vi "测试1005.vi"() -> ()   [LabVIEW 2016]
uses:
  <vilib>/Instr/_visa.llb/VISA Configure Serial Port (Instr).vi
panel:
  out "发送命令 2":string
  in  "暂停 2":bool
  in  "故障腿 2":string(combo)
  in  "控制方法 2":string(combo)
  in  "退化故障 2":string(combo)
  in  "卡滞角度 2":string
  in  "角度（小数） 2":string
  in  "卡滞发生时间 2":string
  in  "小数 2":string
  in  "控制程序启动 2":bool
  in  "复位 2":bool
  out "接受字符串":string
  in  "波特率":dbl
  in  "data bits (8)":u16=8 caption="数据比特(8)" min=5 max=8 step=1
  in  "arduino端口":refnum<visa-resource-name>
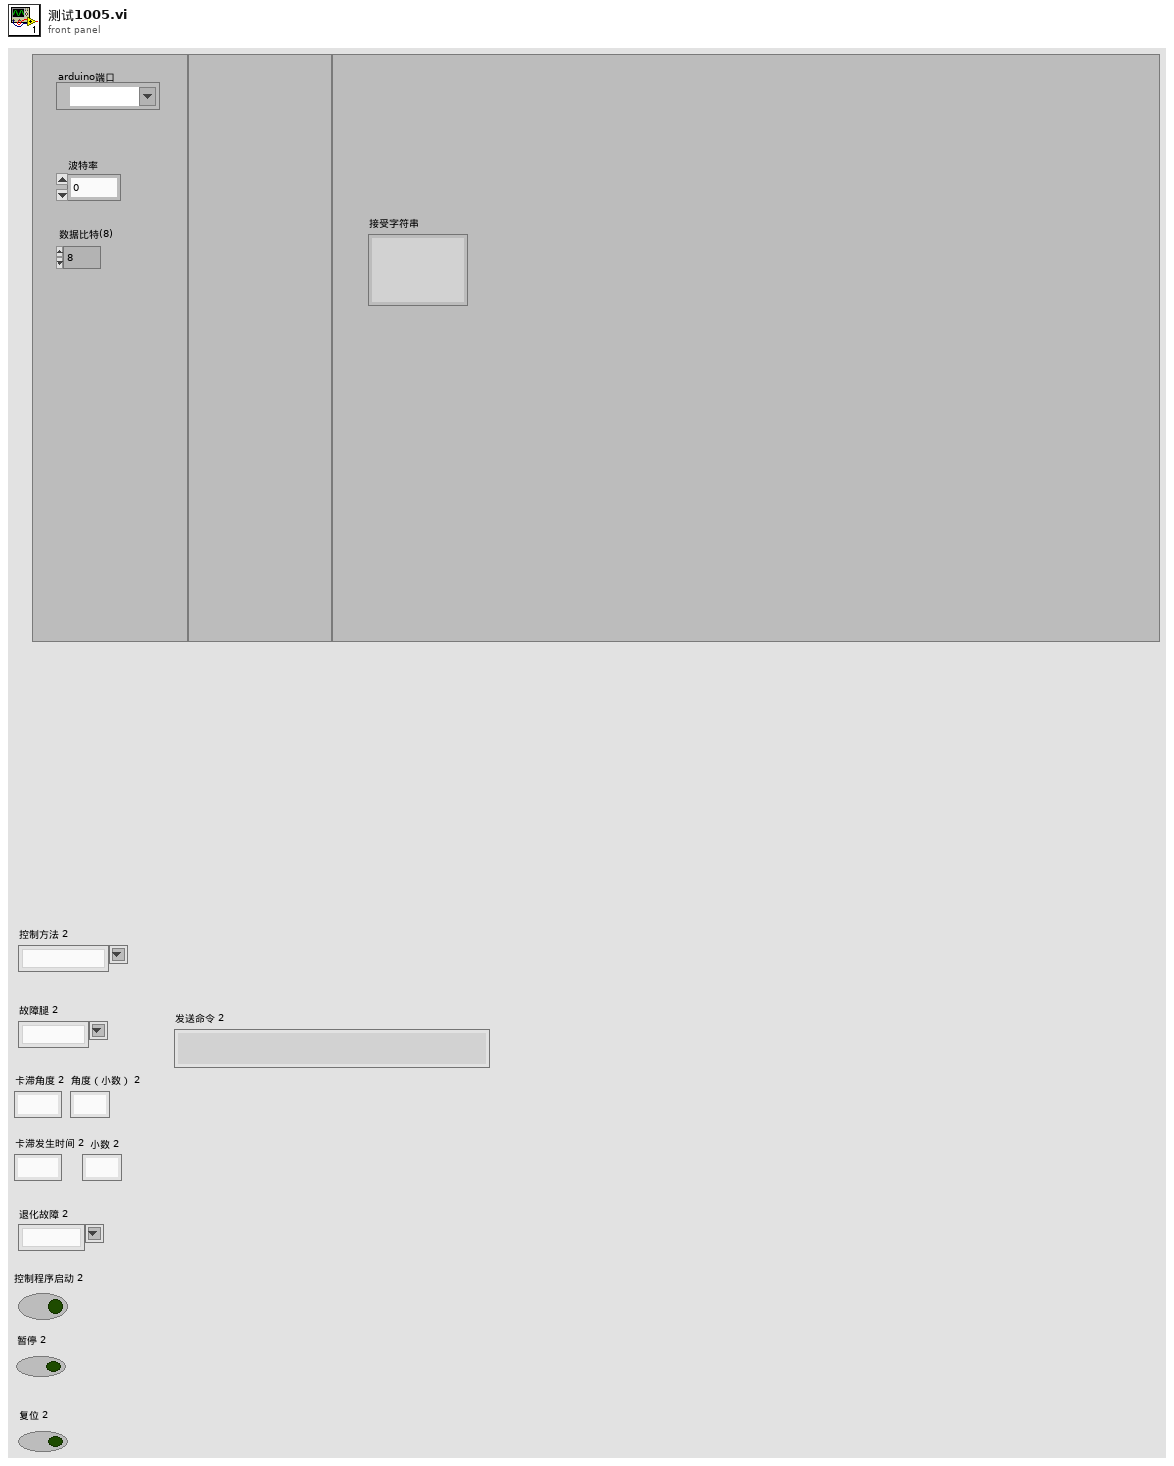
[diagram p1: front panel]
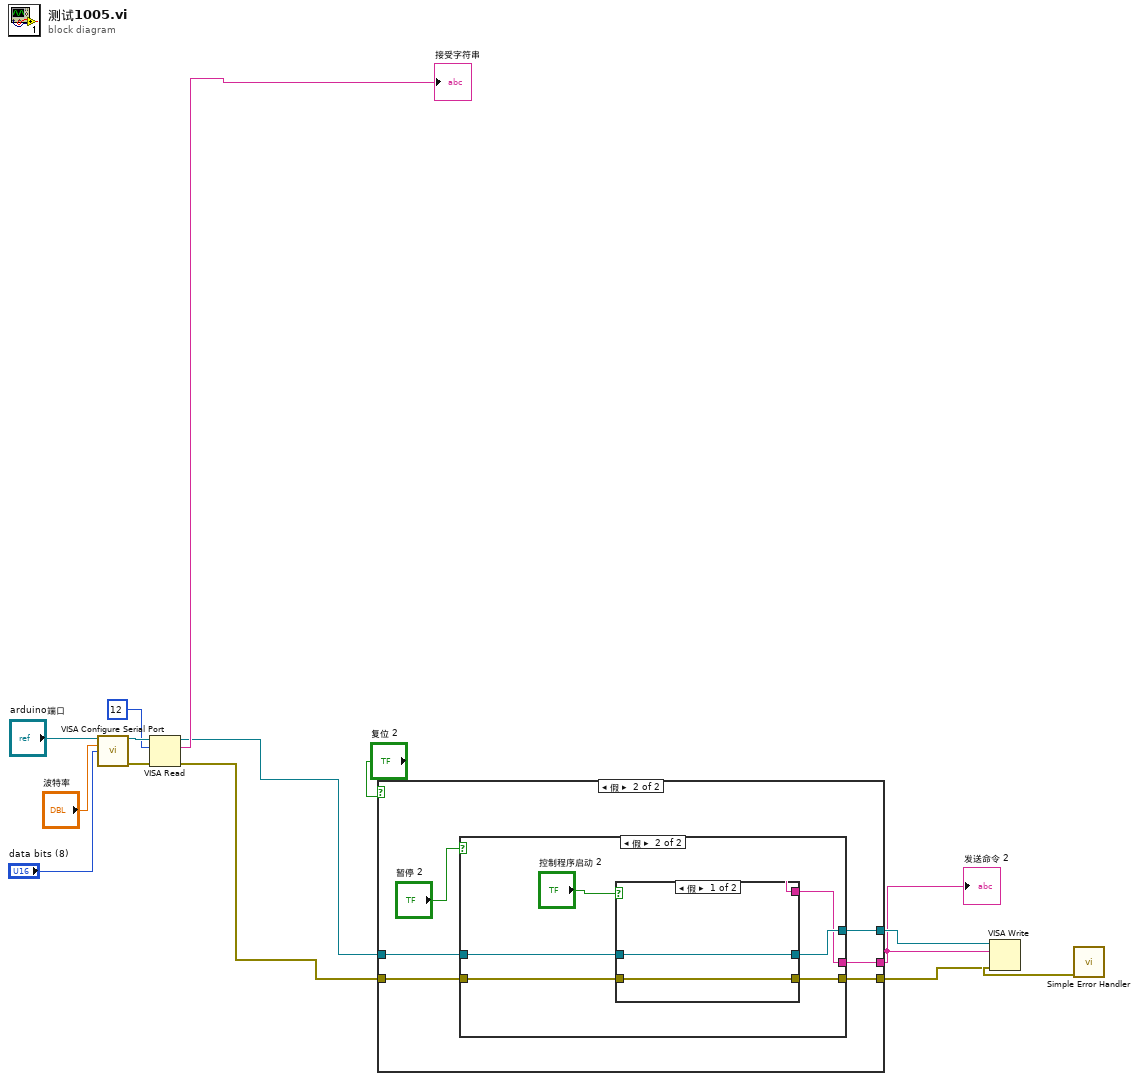
[diagram p0: block diagram]
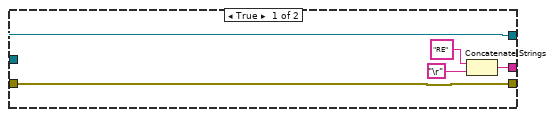
[diagram p2: hidden frame]
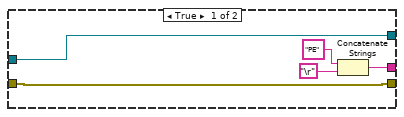
[diagram p3: hidden frame]
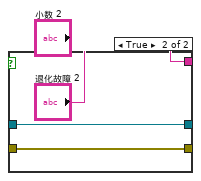
[diagram p4: hidden frame]
diagram:
  n1 = call-poly "VISA Configure Serial Port"("VISA resource name"="arduino端口", "baud rate (9600)"="波特率", "data bits (8)"="data bits (8)") -> ("VISA resource name out"=w11:refnum<visa-resource-name>, "error out"=w9:errorcluster)  [unwired: 11 in]
  n2 = VISA Read(VISA resource name=w11, byte count=12, error in (no error)=w9) -> (VISA resource name out=w1:refnum<visa-resource-name>, read buffer=→"接受字符串":string, error out=w2:errorcluster)  [unwired: 1 out]
  n3 = case shown="假" "复位 2" {
    tunnel: w1 -> [w15 w25]
    tunnel: w2 -> [w16 w24]
    tunnel: [w15 w22] -> w5
    tunnel: [w17 w21] -> w3
    tunnel: [w16 w20] -> w4
    frame True {
      n4 = Concatenate Strings("RE", "\r") -> (w17:string)
    }
    frame False {
      n5 = case shown="假" "暂停 2" {
        tunnel: w25 -> [w28 w36]
        tunnel: w24 -> [w26 w34]
        tunnel: [w28 w33] -> w22
        tunnel: [w27 w32] -> w21
        tunnel: [w26 w31] -> w20
        frame True {
          n6 = Concatenate Strings("PE", "\r") -> (w27:string)
        }
        frame False {
          n7 = case shown="假" "控制程序启动 2" {
            tunnel: w36 -> [w38 w42]
            tunnel: w34 -> [w39 w40]
            tunnel: [w38 w42] -> w33
            tunnel: ["\r" w41] -> w32
            tunnel: [w39 w40] -> w31
            frame False {
            }
            frame True {
              n8 = Concatenate Strings("S", "控制方法 2", "故障腿 2", "卡滞角度 2", "角度（小数） 2", "卡滞发生时间 2", "小数 2", "退化故障 2", "E", "\r") -> (w41:string)
            }
          }
        }
      }
    }
  }
  "发送命令 2" <- w3
  n9 = VISA Write(VISA resource name=w5, write buffer=w3, error in (no error)=w4) -> (error out=w6:errorcluster)  [unwired: 2 out]
  n10 = call <vilib>:"Simple Error Handler.vi"("error in (no error)"=w6) -> ()  [unwired: 1 in, 8 out]
